vi "Execute Correction.vi"(8 "error in (no error)":errorcluster, 9 "Short Correction (T:Yes)":bool=TRUE, 10 "Open Correction (T:Yes)":bool=TRUE, 11 "VISA resource name":refnum<visa-resource-name>) -> (0 "error out":errorcluster, 3 "VISA resource name out":refnum<visa-resource-name>)   [LabVIEW 2016, in "Agilent E4980.lvlib"]
doc: "Executes open and short corrections based on all frequency points."
uses:
  <instrlib>/Agilent E4980/Agilent E4980.lvlib
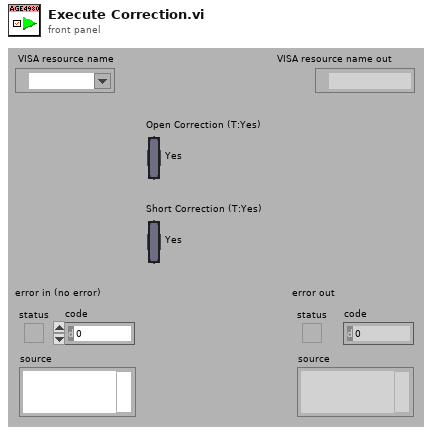
[diagram p1: front panel]
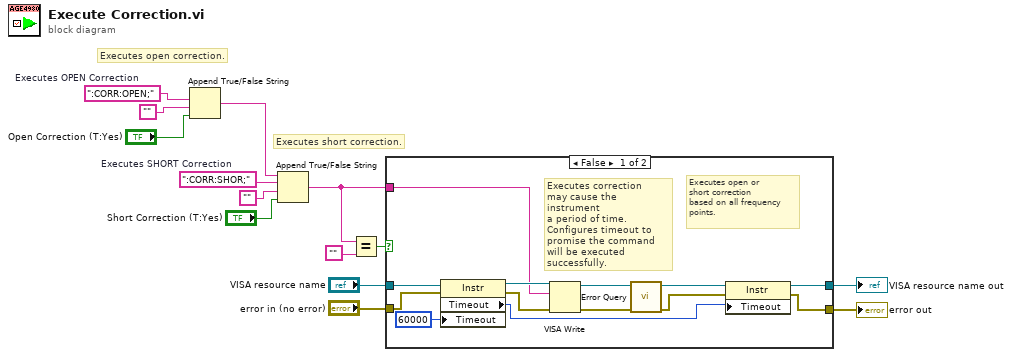
[diagram p0: block diagram]
diagram:
  w11 = ":CORR:SHOR;"  # Executes SHORT Correction
  w14 = ":CORR:OPEN;"  # Executes OPEN Correction
  # "Executes short correction."
  # "Executes open correction."
  n1 = Append True/False String(1:"Open Correction (T:Yes)", 2:"" ("Empty String Constant"), 3:w14) -> (0:w3:string)  [unwired: 1 in]
  n2 = Append True/False String(1:"Short Correction (T:Yes)", 2:"" ("Empty String Constant"), 3:w11, 4:w3) -> (0:w2:string)
  n3 = Equal?(x=w2, y="" ("Empty String Constant")) -> (x = y?=w8:bool)
  n4 = case shown="False" w8 {
    tunnel: "VISA resource name" -> [w27 w29]
    tunnel: "error in (no error)" -> [w26 w28]
    tunnel: [w16 w29] -> w5
    tunnel: [w15 w28] -> w4
    tunnel: w2 -> [w22 _]
    frame False {
      # "Executes correction\nmay cause the instrument\na period of time.\nConfigures timeout to\npromise the command\nwill be executed\nsuccessfully."
      # "Executes open or\nshort correction\nbased on all frequency\npoints."
      n5 = property on="Property Node" class="Instr"(reference=w27, error in=w26, "Timeout"=u32 60000 ("General Settings:Timeout Value")) -> (reference out=w24:refnum<visa-resource-name>, error out=w23:errorcluster, "Timeout"=w17:u32)
      n6 = VISA Write(VISA resource name=w24, write buffer=w22, error in (no error)=w23) -> (VISA resource name out=w21:refnum<visa-resource-name>, error out=w20:errorcluster)  [unwired: 1 out]
      n7 = call <instrlib>:"Error Query.vi"("error in (no error)"=w20, "VISA resource name"=w21) -> ("error out"=w18:errorcluster, "VISA resource name out"=w19:refnum<visa-resource-name>)  [unwired: 6 in, 2 out]
      n8 = property on="Property Node" class="Instr"(reference=w19, error in=w18, "Timeout"=w17) -> (reference out=w16:refnum<visa-resource-name>, error out=w15:errorcluster)
    }
    frame True {
      # "Doesn't send anything\nto the instrument."
    }
  }
  "error out" <- w4
  "VISA resource name out" <- w5
